vi "Configure Trigger (Ethernet - MAC).vi"(0 "VISA resource name":refnum<visa-resource-name>, 1 "Upper Length (\"XXXXXXX\")":string="XXXXXXX", 5 "Trigger Source (9: Bus 1)":u16(ring)=9 items=["Bus 1"=9, "Bus 2"=10], 7 "Source Address  (\"XXXXXXX\")":string="XXXXXXX", 9 "Destination Address  (\"XXXXXXX\")":string="XXXXXXX", 11 "error in (no error)":errorcluster, 12 "Length (\"XXXXXXX\")":string="XXXXXXX") -> (4 "VISA resource name out":refnum<visa-resource-name>, 15 "error out":errorcluster)   [LabVIEW 2013, in "Tektronix DPO MSO 2000 4000 Series.lvlib"]
doc: "Configures MAC trigger settings for Ethernet trigger. \n\n<B>Note:</B>\nThis VI only applies to DPO4034B, DPO4054B, DPO4104B, MSO4034B, MSO4054B, MSO4104B."
uses:
  Tektronix DPO MSO 2000 4000 Series.lvlib
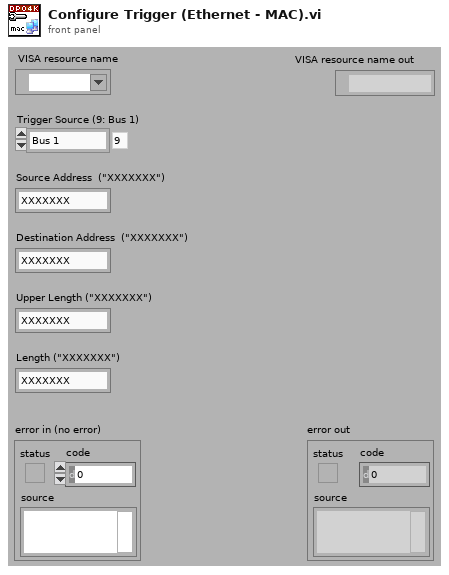
[diagram p1: front panel]
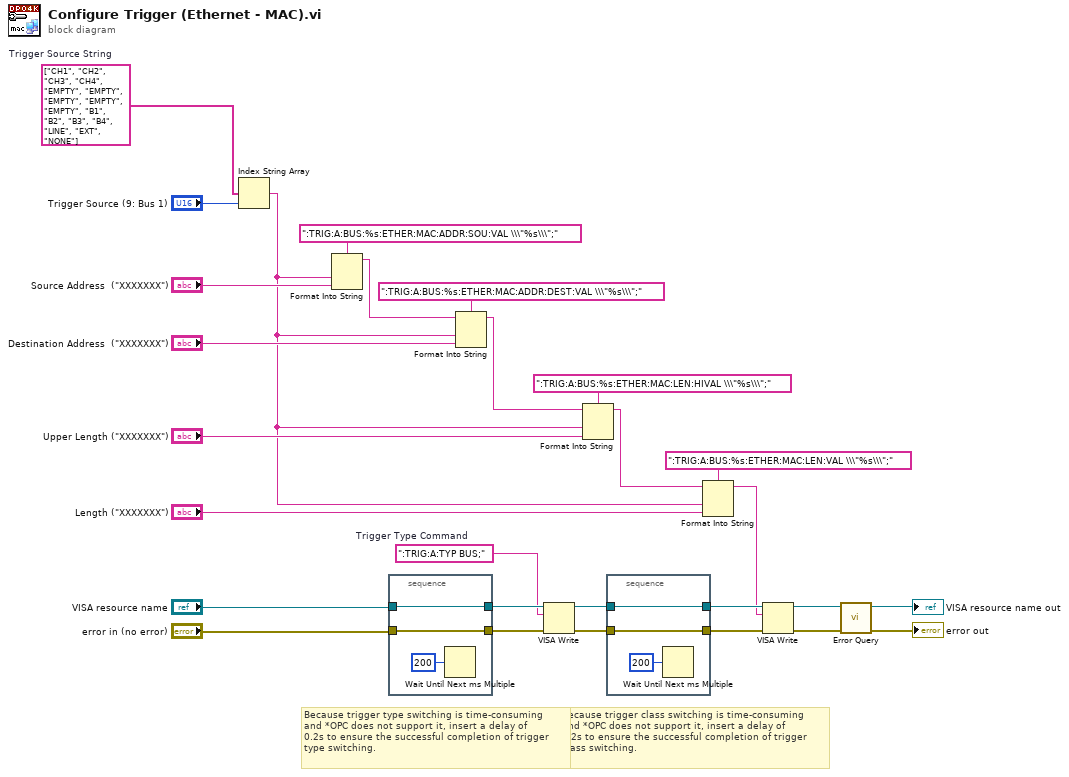
[diagram p0: block diagram]
diagram:
  w21 = string[] ["CH1", "CH2", "CH3", "CH4", "EMPTY", "EMPTY", "EMPTY", "EMPTY", "EMPTY", "B1", "B2", "B3", "B4", "LINE", "EXT", "NONE"]  # Trigger Source String
  w26 = ":TRIG:A:TYP BUS;"  # Trigger Type Command
  # "Because trigger class switching is time-consuming\nand *OPC does not support it, insert a delay of\n0.2s to ensure the successful completion of trigger\nclass switching."
  # "Because trigger type switching is time-consuming\nand *OPC does not support it, insert a delay of\n0.2s to ensure the successful completion of trigger\ntype switching."
  n1 = Index String Array(1:"Trigger Source (9: Bus 1)", 2:w21) -> (0:w2:string)  [unwired: 1 in]
  n2 = Format Into String(format string=":TRIG:A:BUS:%s:ETHER:MAC:ADDR:SOU:VAL \\\"%s\\\";", w2, "Source Address  (\"XXXXXXX\")") -> (resulting string=w9:string)  [unwired: 2 in, 1 out]
  n3 = stacked-sequence {
    tunnel: "VISA resource name" -> [w30]
    tunnel: [w30] -> w28
    tunnel: "error in (no error)" -> [w29]
    tunnel: [w29] -> w27
    frame #0 {
      n4 = Wait Until Next ms Multiple(millisecond multiple=u32 200) -> ()  [unwired: 1 out]
    }
  }
  n5 = Format Into String(format string=":TRIG:A:BUS:%s:ETHER:MAC:ADDR:DEST:VAL \\\"%s\\\";", initial string=w9, w2, "Destination Address  (\"XXXXXXX\")") -> (resulting string=w4:string)  [unwired: 1 in, 1 out]
  n6 = VISA Write(VISA resource name=w28, write buffer=w26, error in (no error)=w27) -> (VISA resource name out=w25:refnum<visa-resource-name>, error out=w24:errorcluster)  [unwired: 1 out]
  n7 = Format Into String(format string=":TRIG:A:BUS:%s:ETHER:MAC:LEN:HIVAL \\\"%s\\\";", initial string=w4, w2, "Upper Length (\"XXXXXXX\")") -> (resulting string=w1:string)  [unwired: 1 in, 1 out]
  n8 = stacked-sequence {
    tunnel: w25 -> [w33]
    tunnel: [w33] -> w23
    tunnel: w24 -> [w32]
    tunnel: [w32] -> w22
    frame #0 {
      n9 = Wait Until Next ms Multiple(millisecond multiple=u32 200) -> ()  [unwired: 1 out]
    }
  }
  n10 = Format Into String(format string=":TRIG:A:BUS:%s:ETHER:MAC:LEN:VAL \\\"%s\\\";", initial string=w1, w2, "Length (\"XXXXXXX\")") -> (resulting string=w3:string)  [unwired: 1 in, 1 out]
  n11 = VISA Write(VISA resource name=w23, write buffer=w3, error in (no error)=w22) -> (VISA resource name out=w19:refnum<visa-resource-name>, error out=w18:errorcluster)  [unwired: 1 out]
  n12 = call "Error Query.vi"("error in (no error)"=w18, "VISA resource name"=w19) -> ("error out"=→"error out":errorcluster, "VISA resource name out"=→"VISA resource name out":refnum<visa-resource-name>)  [unwired: 6 in, 2 out]
